vi "Execution_Appli_ReadNIFileAndSetAppGenSettingsCluster.vi"(8 "error in":errorcluster, 11 "INI Path":path) -> (0 "error out":errorcluster, 2 "GenericSettings":T1)   [LabVIEW 2013, in "EVE.lvclass"]
uses:
  EVE.lvclass
  App_GenericSettings.ctl
  <vilib>/Utility/config.llb/Read Key (Boolean).vi
  <vilib>/Utility/config.llb/Read Key (Path).vi
  <vilib>/Utility/config.llb/Read Key (String).vi
  <vilib>/Utility/config.llb/Read Key (Double).vi
  <vilib>/Utility/config.llb/Read Key (I32).vi
  <vilib>/Utility/config.llb/NI_LVConfig.lvlib
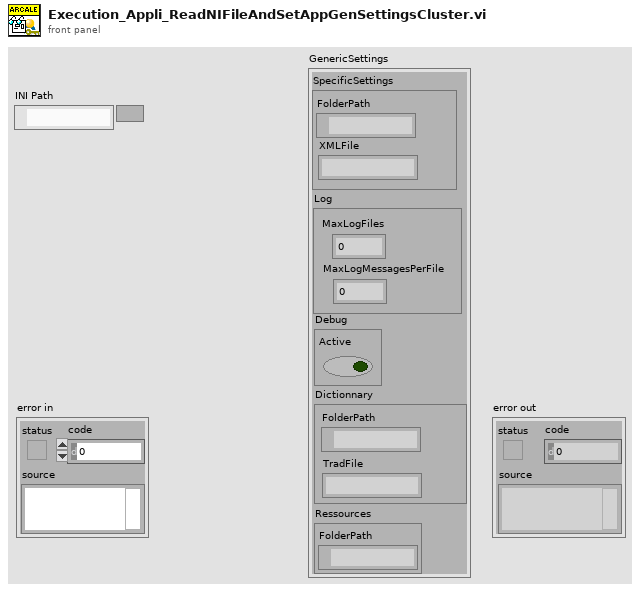
[diagram p1: front panel]
types:
  T1 = typedef "EVE.lvclass/App_GenericSettings.ctl" = cluster{"SpecificSettings":cluster{"FolderPath":path, "XMLFile":string}, "Log":cluster{"MaxLogFiles":i32, "MaxLogMessagesPerFile":i32}, "Debug":cluster{"Active":bool}, "Dictionnary":cluster{"FolderPath":path, "TradFile":string}, "Ressources":cluster{"FolderPath":path}}
  T2 = typedef "NI_LVConfig.lvlib/Config Data RefNum.ctl" = refnum<k1>
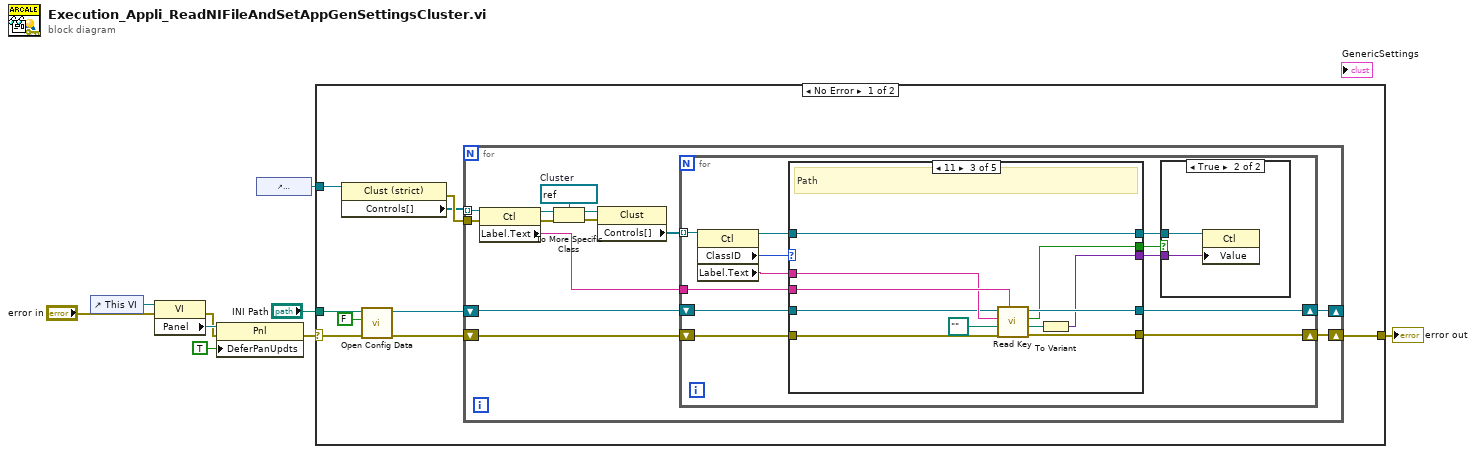
[diagram p0: block diagram]
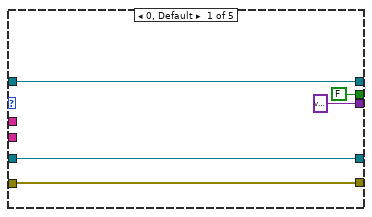
[diagram p3: hidden frame]
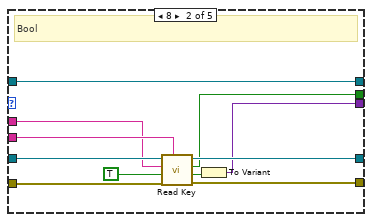
[diagram p4: hidden frame]
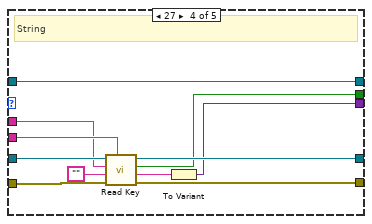
[diagram p5: hidden frame]
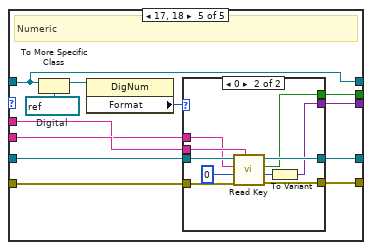
[diagram p6: hidden frame]
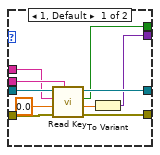
[diagram p7: hidden frame]
diagram:
  n1 = control-ref of="This VI"() -> (w6:refnum<vi>)
  n2 = property class="VI"(reference=w6, error in="error in") -> (error out=w2:errorcluster, "Panel"=w5:refnum<vi>)  [unwired: 1 out]
  n3 = property class="Pnl"(reference=w5, error in=w2, "DeferPanUpdts"=TRUE ("Defer Panel Updates")) -> (error out=w1:errorcluster)  [unwired: 1 out]
  n4 = control-ref of="GenericSettings"() -> (w7:refnum<vi>)
  n5 = case shown="No Error" w1 {
    selector: w1 -> [w18 w116]
    tunnel: [w10 w116] -> w9
    tunnel: "INI Path" -> [w17 _]
    tunnel: w7 -> [w15 _]
    frame No Error {
      n6 = property class="Clust (strict)"(reference=w15) -> (error out=w14:errorcluster, "Controls[]"=w13:refnum<vi>[])  [unwired: 1 in, 1 out]
      n7 = call <vilib>:"Open Config Data.vi"("error in (no error)"=w18, "create file if necessary (T)"=FALSE, "configuration file path"=w17) -> ("error out"=w11:errorcluster, "refnum"=w12:T2)  [unwired: 6 in, 1 out]
      n8 = for {
        tunnel: w13 -> [w29] mode=indexing
        shift-right: [w20] -> w10
        shift-left: w11 -> [w31]
        tunnel: w14 -> [w22]
        shift-right: [w19] -> _
        shift-left: w12 -> [w30]
        w26 = refnum<vi> refnum  # Cluster
        n9 = property class="Ctl"(reference=w29, error in=w22) -> (reference out=w28:refnum<vi>, error out=w23:errorcluster, "Label.Text"=w27:string)
        n10 = To More Specific Class(target class=w26, reference=w28, error in=w23) -> (specific class reference=w25:refnum<vi>, error out=w24:errorcluster)
        n11 = property class="Clust"(reference=w25, error in=w24) -> ("Controls[]"=w21:refnum<vi>[])  [unwired: 2 out]
        n12 = for {
          tunnel: w27 -> [w41]
          tunnel: w21 -> [w40] mode=indexing
          shift-right: [w37] -> w20
          shift-left: w31 -> [w43]
          shift-right: [w35] -> w19
          shift-left: w30 -> [w42]
          n13 = property class="Ctl"(reference=w40) -> (reference out=w36:refnum<vi>, "ClassID"=w38:u32, "Label.Text"=w39:string)  [unwired: 1 in, 1 out]
          n14 = case shown="11" w38 {
            tunnel: w43 -> [w50 w58 w70 w78 w92]
            tunnel: w42 -> [w49 w61 w68 w83 w95]
            tunnel: w41 -> [_ w60 w72 w82 w94]
            tunnel: w39 -> [_ w59 w71 w81 w93]
            tunnel: [w50 w56 w69 w80 w91] -> w37
            tunnel: w36 -> [w48 w54 w62 w74 w85]
            tunnel: [w49 w55 w67 w79 w87] -> w35
            tunnel: [variant ("Variant") w52 w63 w75 w84] -> w32
            tunnel: [w48 w54 w62 w74 w85] -> w33
            tunnel: [FALSE ("found?") w51 w64 w73 w86] -> w34
            frame 0, Default {
            }
            frame 8 {
              # "Bool"
              n15 = call-poly <vilib>:"Read Key.vi"("section"=w60, "error in (no error)"=w58, "default value"=TRUE, "key"=w59, "refnum"=w61) -> ("error out"=w56:errorcluster, "value"=w53:bool, "found?"=w51:bool, "refnum out"=w55:T2)  [unwired: 3 in]
              n16 = To Variant(anything=w53) -> (Variant=w52:variant)
            }
            frame 11 {
              # "Path"
              n17 = call-poly <vilib>:"Read Key.vi"("section"=w72, "error in (no error)"=w70, "default value"=path "", "key"=w71, "refnum"=w68) -> ("error out"=w69:errorcluster, "value"=w65:path, "found?"=w64:bool, "refnum out"=w67:T2)  [unwired: 3 in]
              n18 = To Variant(anything=w65) -> (Variant=w63:variant)
            }
            frame 27 {
              # "String"
              n19 = call-poly <vilib>:"Read Key.vi"("section"=w82, "error in (no error)"=w78, "default value"="", "key"=w81, "refnum"=w83) -> ("error out"=w80:errorcluster, "value"=w76:string, "found?"=w73:bool, "refnum out"=w79:T2)  [unwired: 3 in]
              n20 = To Variant(anything=w76) -> (Variant=w75:variant)
            }
            frame 17, 18 {
              w89 = refnum<vi> refnum  # Digital
              # "Numeric"
              n21 = To More Specific Class(target class=w89, reference=w85) -> (specific class reference=w90:refnum<vi>)  [unwired: 1 in, 1 out]
              n22 = property class="DigNum"(reference=w90) -> ("Format"=w88:u8)  [unwired: 1 in, 2 out]
              n23 = case shown="0" w88 {
                tunnel: w95 -> [w105 w115]
                tunnel: w94 -> [w104 w114]
                tunnel: w93 -> [w103 w113]
                tunnel: w92 -> [w100 w110]
                tunnel: [w102 w112] -> w91
                tunnel: [w101 w111] -> w87
                tunnel: [w98 w108] -> w86
                tunnel: [w96 w106] -> w84
                frame 1, Default {
                  n24 = call-poly <vilib>:"Read Key.vi"("section"=w104, "error in (no error)"=w100, "default value"=0.0, "key"=w103, "refnum"=w105) -> ("error out"=w102:errorcluster, "value"=w97:dbl, "found?"=w98:bool, "refnum out"=w101:T2)  [unwired: 3 in]
                  n25 = To Variant(anything=w97) -> (Variant=w96:variant)
                }
                frame 0 {
                  n26 = call-poly <vilib>:"Read Key.vi"("section"=w114, "error in (no error)"=w110, "default value"=0, "key"=w113, "refnum"=w115) -> ("error out"=w112:errorcluster, "value"=w107:i32, "found?"=w108:bool, "refnum out"=w111:T2)  [unwired: 3 in]
                  n27 = To Variant(anything=w107) -> (Variant=w106:variant)
                }
              }
            }
          }
          n28 = case shown="True" w34 {
            tunnel: w33 -> [_ w45]
            tunnel: w32 -> [_ w44]
            frame False {
            }
            frame True {
              n29 = property class="Ctl"(reference=w45, "Value"=w44) -> ()  [unwired: 1 in, 2 out]
            }
          }
        }
      }
    }
    frame Error {
    }
  }
  "error out" <- w9
